vi "Next Button Facade.vi"(0 "Data In":T4, 2 "Display State In":T2, 3 "Container State":T3) -> (6 "Data Out":T4, 7 "Display State Out":T2, 8 "Action":T1)   [LabVIEW 2010, in "Next Button (Modern).xctl"]
uses:
  <vilib>/Navigation Controls/Next Button/Next Button (Modern).xctl
  <vilib>/Navigation Controls/Next Button/Next Button Data.ctl
  <vilib>/_xctls/Container State.ctl
  <vilib>/Navigation Controls/Next Button/Next Button State.ctl
  <vilib>/_xctls/Action.ctl
  <vilib>/_xctls/XControlSupport.lvlib
  <vilib>/Navigation Controls/NI_Navigation.lvlib
panel:
  out "Error":bool
  in  "Next Button":bool
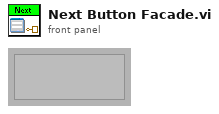
[diagram p1: front panel]
types:
  T1 = typedef "XControlSupport.lvlib/Action.ctl" = cluster{"Data Changed?":bool, "State Changed?":bool, "Action Name":string}
  T2 = typedef "Next Button (Modern).xctl/Next Button State.ctl" = cluster{"Button Text":string}
  T3 = typedef "XControlSupport.lvlib/Container State.ctl" = cluster{"Indicator?":bool, "Run Mode?":bool, " Refnum":refnum<vi>}
  T4 = typedef "Next Button (Modern).xctl/Next Button Data.ctl" = bool
  T5 = enum32{"Invalid", "Standard", "Closed", "Hidden", "Minimized", "Maximized"}
  T6 = enum32{"Bad", "Idle", "Run top level", "Running"}
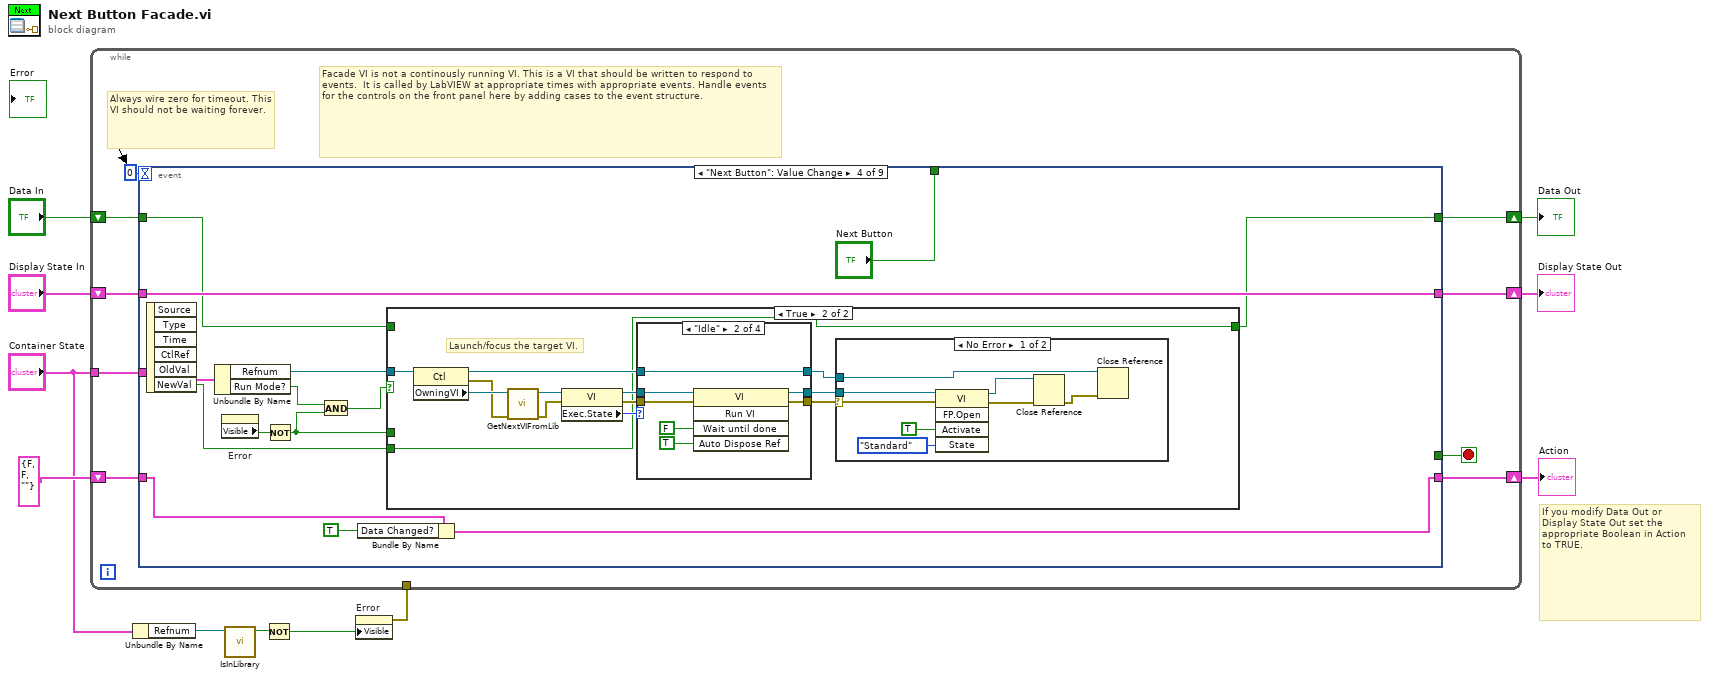
[diagram p0: block diagram]
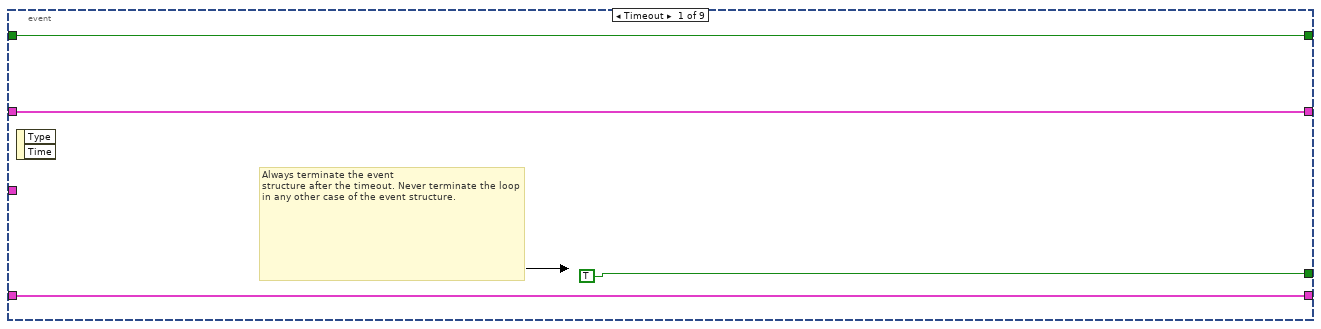
[diagram p2: hidden frame]
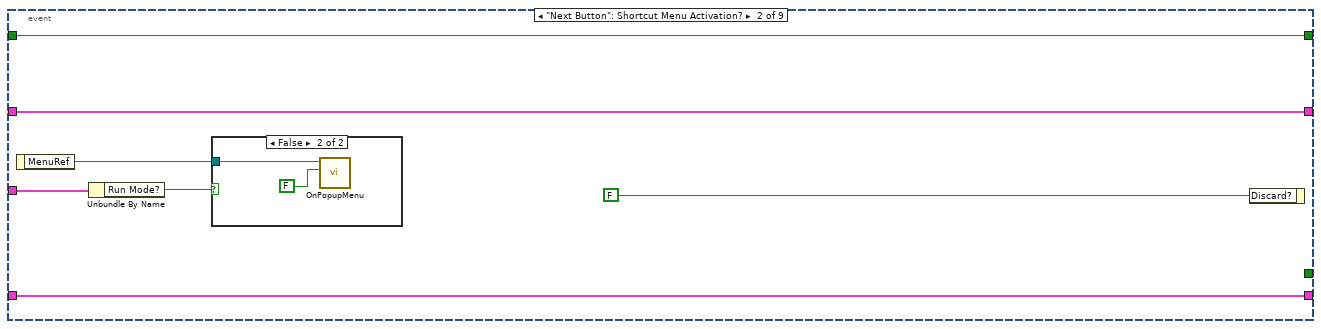
[diagram p3: hidden frame]
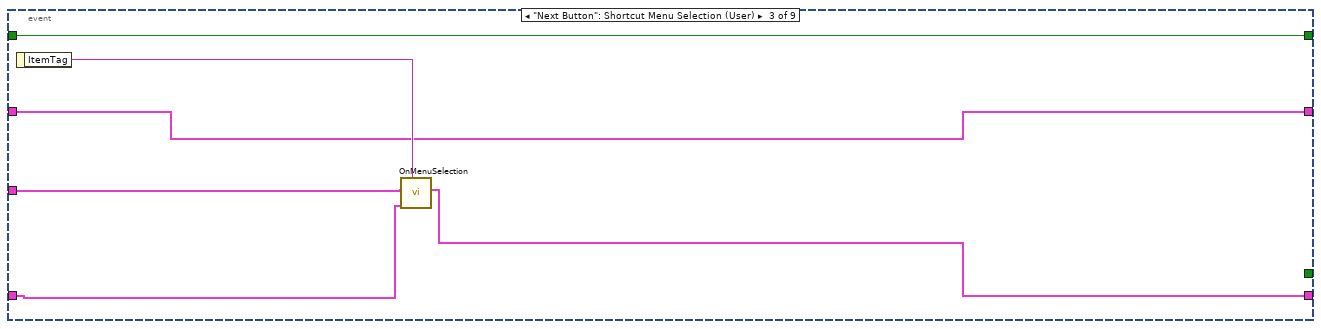
[diagram p5: hidden frame]
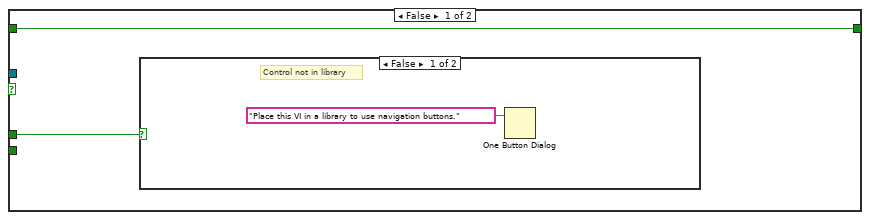
[diagram p6: hidden frame]
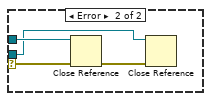
[diagram p8: hidden frame]
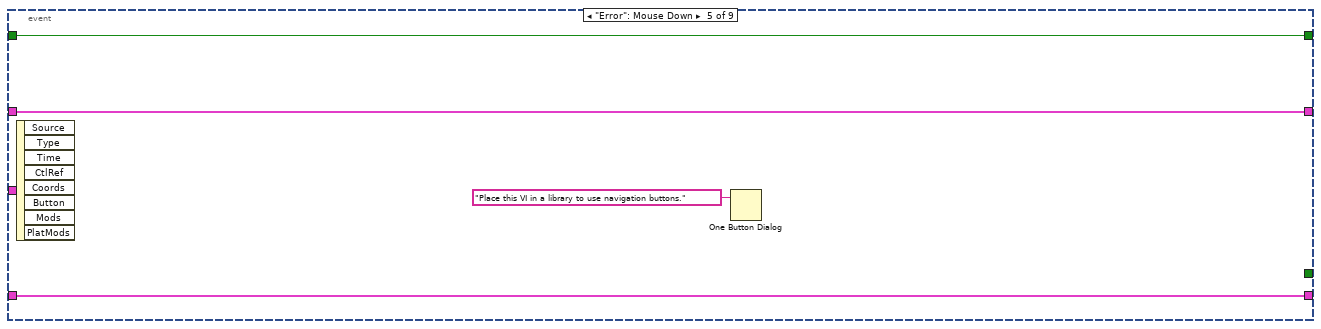
[diagram p12: hidden frame]
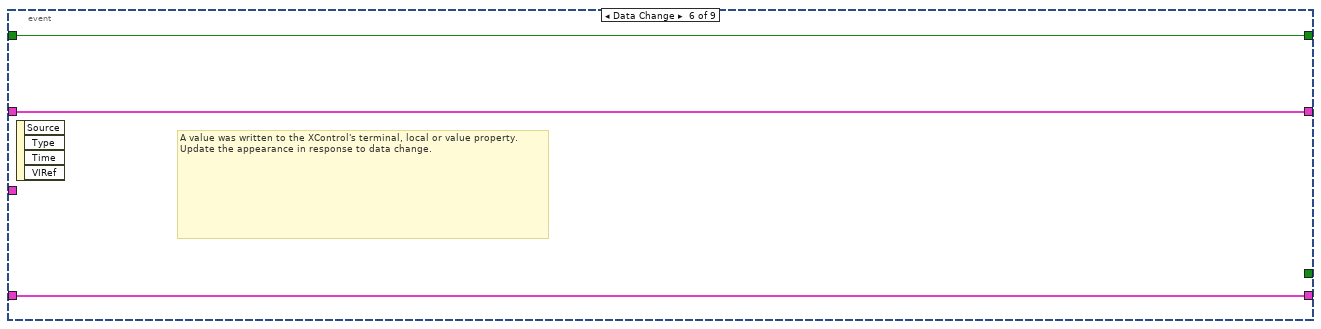
[diagram p13: hidden frame]
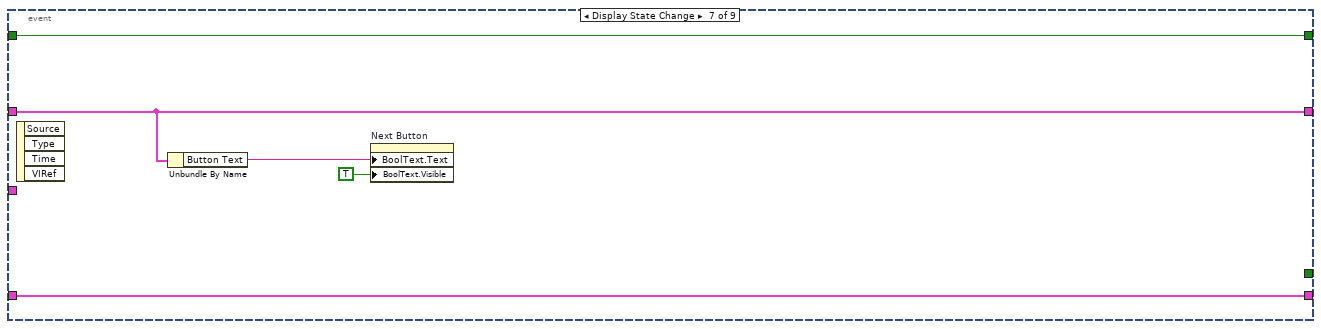
[diagram p14: hidden frame]
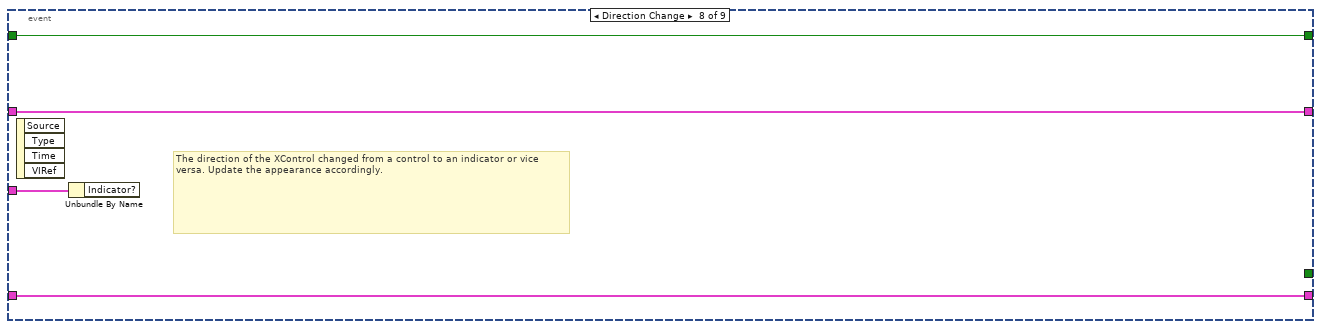
[diagram p15: hidden frame]
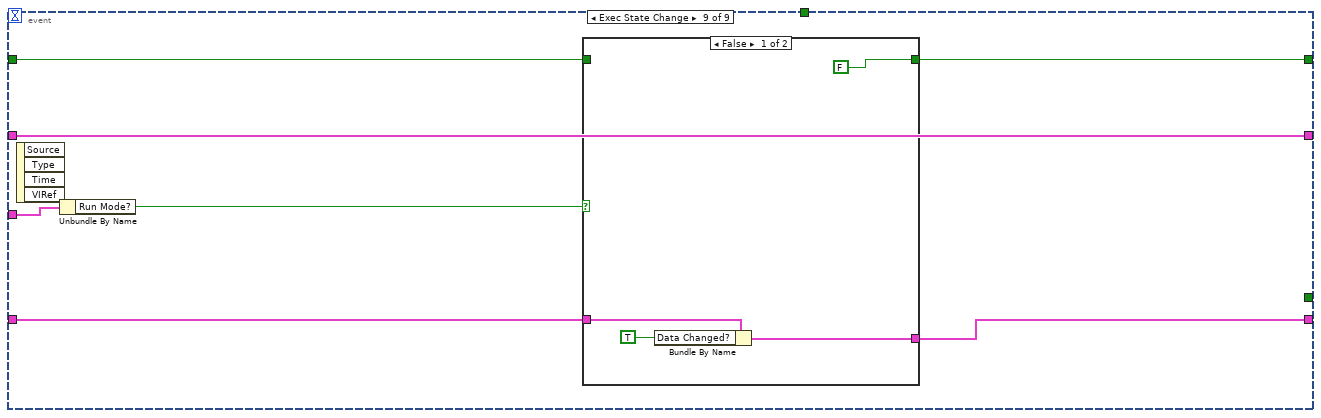
[diagram p16: hidden frame]
diagram:
  # "If you modify Data Out or\nDisplay State Out set the\nappropriate Boolean in Action\nto TRUE."
  n1 = Unbundle By Name("Container State") -> ("Refnum"=w5:refnum<vi>)
  n2 = call <vilib>:"IsInLibrary.vi"("Control refnum"=w5) -> ("In library?"=w4:bool)  [unwired: 10 out]
  n3 = Not(x=w4) -> (.not. x?=w3:bool)
  n4 = property on="Error" class="Bool (strict)"("Visible"=w3) -> (error out=w1:errorcluster)  [unwired: 2 in, 1 out]
  n5 = while {
    shift-right: [w19] -> w9
    shift-left: "Display State In" -> [w20]
    tunnel: "Container State" -> [w16]
    shift-right: [w14] -> w11
    shift-left: "Data In" -> [w15]
    shift-right: [w12] -> w7
    shift-left: T1 {"Data Changed?"=FALSE, "State Changed?"=FALSE, "Action Name"=""} ("Action") -> [w13]
    tunnel: w1 -> [_]
    stop <- w18 stop-if-true
    # "Facade VI is not a continously running VI. This is a VI that should be written to respond to events.  It is called by LabVIEW at appropriate times with appropriate events. Handle events for the controls on the front panel here by adding cases to the event structure."
    # "Always wire zero for timeout. This\nVI should not be waiting forever."
    n6 = event shown="[3] \"Next Button\": Value Change" {
      selector: _ -> [_ _ _ _ _ _ _ _ _]
      dyn-events: _ -> [_ _ _ _ _ _ _ _ _]
      timeout: 0 -> [_ _ _ _ _ _ _ _ _]
      tunnel: w20 -> [w22 w30 w36 w53 w100 w103 w107 w112 w115]
      tunnel: [w22 w30 w36 w53 w100 w103 w107 w112 w115] -> w19
      tunnel: [TRUE _ _ _ _ _ _ _ _] -> w18
      tunnel: w16 -> [_ w28 w37 w49 _ _ _ w113 w120]
      tunnel: w15 -> [w21 w31 w39 w46 w101 w104 w109 w111 w116]
      tunnel: [w21 w31 w39 w44 w101 w104 w109 w111 w118] -> w14
      tunnel: [w23 w29 w34 w51 w99 w102 w108 w110 w117] -> w12
      tunnel: w13 -> [w23 w29 w35 w52 w99 w102 w108 w110 w114]
      tunnel: [_ _ _ "Next Button" _ _ _ _ _] -> _
      event Timeout {
        # "Always terminate the event\nstructure after the timeout. Never terminate the loop in any other case of the event structure."
        n7 = event-data() -> ()  [unwired: 1 in, 2 out]
      }
      event "Next Button": Shortcut Menu Activation? {
        n8 = event-data() -> ("MenuRef"=w26:refnum<k9>)  [unwired: 1 in]
        n9 = Unbundle By Name(w28) -> ("Run Mode?"=w25:bool)
        n10 = case shown="False" w25 {
          tunnel: w26 -> [_ w33]
          frame True {
          }
          frame False {
            n11 = call <vilib>:"OnPopupMenu.vi"("Configurable?"=FALSE, "MenuRef"=w33) -> ()  [unwired: 10 in]
          }
        }
        n12 = event-data("Discard?"=FALSE) -> ()  [unwired: 1 in, 1 out]
      }
      event "Next Button": Shortcut Menu Selection (User) {
        n13 = event-data() -> ("ItemTag"=w38:string)  [unwired: 1 in]
        n14 = call <vilib>:"OnMenuSelection.vi"("Tag"=w38, "Action In"=w35, "Container State"=w37) -> ("Action Out"=w34:T1)  [unwired: 7 in, 1 out]
      }
      event "Next Button": Value Change {
        n15 = event-data() -> ("NewVal"=w45:bool)  [unwired: 1 in, 5 out]
        n16 = Unbundle By Name(w49) -> ("Refnum"=w48:refnum<vi>, "Run Mode?"=w42:bool)
        n17 = property on="Error" class="Bool (strict)"() -> ("Visible"=w43:bool)  [unwired: 2 in, 2 out]
        n18 = Not(x=w43) -> (.not. x?=w40:bool)
        n19 = And(x=w42, y=w40) -> (x .and. y?=w41:bool)
        n20 = Bundle By Name(cluster=w52, "Data Changed?"=TRUE) -> (w51:T1)
        n21 = case shown="True" w41 {
          tunnel: w48 -> [_ w69]
          tunnel: w46 -> [w55 _]
          tunnel: w45 -> [_ w57]
          tunnel: [w55 w57] -> w44
          tunnel: w40 -> [w54 _]
          frame False {
            n22 = case shown="False" w54 {
              frame False {
                # "Control not in library"
                n23 = One Button Dialog(message="Place this VI in a library to use navigation buttons.") -> ()  [unwired: 1 in, 1 out]
              }
              frame True {
                # "No problems"
              }
            }
          }
          frame True {
            # "Launch/focus the target VI."
            n24 = property class="Ctl"(reference=w69) -> (reference out=w59:refnum<vi>, error out=w67:errorcluster, "OwningVI"=w68:refnum<vi>)  [unwired: 1 in]
            n25 = call <vilib>:"GetNextVIFromLib.vi"("error in (no error)"=w67, "VI Reference"=w68) -> ("error out"=w65:errorcluster, "Next VI"=w66:refnum<vi>)  [unwired: 8 out]
            n26 = property class="VI"(reference=w66, error in=w65) -> (reference out=w62:refnum<vi>, error out=w63:errorcluster, "Exec.State"=w64:T6)
            n27 = case shown="\"Idle\"" w64 {
              tunnel: w63 -> [w83 w91 w93 w97]
              tunnel: w62 -> [w84 w90 w94 w96]
              tunnel: [w83 w87 w93 w97] -> w60
              tunnel: [w84 w86 w94 w96] -> w61
              tunnel: w59 -> [w82 w85 w92 w95]
              tunnel: [w82 w85 w92 w95] -> w58
              frame "Bad", Default {
              }
              frame "Idle" {
                n28 = invoke class="VI" method="Run VI"(reference=w90, error in=w91, "Wait until done"=FALSE ("Wait Until Done"), "Auto Dispose Ref"=TRUE ("Auto Dispose Reference")) -> (reference out=w86:refnum<vi>, error out=w87:errorcluster)  [unwired: 1 in, 3 out]
              }
              frame "Run top level" {
              }
              frame "Running" {
              }
            }
            n29 = case shown="No Error" w60 {
              selector: w60 -> [w76 w80]
              tunnel: w61 -> [w77 w78]
              tunnel: w58 -> [w73 w81]
              frame No Error {
                n30 = invoke class="VI" method="FP.Open"(reference=w77, error in=w76, "Activate"=TRUE ("Activate?"), "State"=T5."Standard") -> (reference out=w72:refnum<vi>, error out=w71:errorcluster)  [unwired: 1 in, 3 out]
                n31 = Close Reference(reference=w72, error in (no error)=w71) -> (error out=w70:errorcluster)
                n32 = Close Reference(reference=w73, error in (no error)=w70) -> ()  [unwired: 1 out]
              }
              frame Error {
                n33 = Close Reference(reference=w81, error in (no error)=w80) -> (error out=w79:errorcluster)
                n34 = Close Reference(reference=w78, error in (no error)=w79) -> ()  [unwired: 1 out]
              }
            }
          }
        }
      }
      event "Error": Mouse Down {
        n35 = event-data() -> ()  [unwired: 1 in, 8 out]
        n36 = One Button Dialog(message="Place this VI in a library to use navigation buttons.") -> ()  [unwired: 1 in, 1 out]
      }
      event Data Change {
        # "A value was written to the XControl's terminal, local or value property.\nUpdate the appearance in response to data change."
        n37 = event-data() -> ()  [unwired: 1 in, 4 out]
      }
      event Display State Change {
        n38 = event-data() -> ()  [unwired: 1 in, 4 out]
        n39 = Unbundle By Name(w107) -> ("Button Text"=w105:string)
        n40 = property on="Next Button" class="Bool"("BoolText.Text"=w105, "BoolText.Visible"=TRUE ("Boolean Text.Visible")) -> ()  [unwired: 2 in, 2 out]
      }
      event Direction Change {
        # "The direction of the XControl changed from a control to an indicator or vice versa. Update the appearance accordingly."
        n41 = event-data() -> ()  [unwired: 1 in, 4 out]
        n42 = Unbundle By Name(w113) -> ()  [unwired: 1 out]
      }
      event Exec State Change {
        n43 = event-data() -> ()  [unwired: 1 in, 4 out]
        n44 = Unbundle By Name(w120) -> ("Run Mode?"=w119:bool)
        n45 = case shown="False" w119 {
          tunnel: [T4 FALSE ("Data In") w125] -> w118
          tunnel: w114 -> [w123 w126]
          tunnel: [w121 w126] -> w117
          tunnel: w116 -> [_ w125]
          frame False {
            n46 = Bundle By Name(cluster=w123, "Data Changed?"=TRUE) -> (w121:T1)
          }
          frame True {
          }
        }
      }
    }
  }
  "Display State Out" <- w9
  "Data Out" <- w11
  "Action" <- w7
